vi "Position Heading.vi"(10 "To":T2, 11 "From":T2) -> (2 "Same Position?":bool, 3 "Heading":T1)   [LabVIEW 2020, in "SquareBattle.lvlib"]
doc: "Returns the closest direction enumeration value from the specified From position to the specied To position. This can be used to more easily move towards a goal position.\n\nIf Same Position? returns True, then the To and From positions are the same and the Heading output will be invalid."
uses:
  SquareBattle.lvlib
  Position.ctl
  Direction.ctl
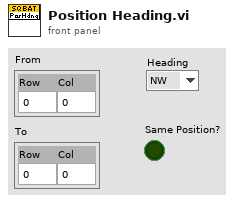
[diagram p1: front panel]
types:
  T1 = typedef "SquareBattle.lvlib/Direction.ctl" = enum16{"NW", "N", "NE", "E", "SE", "S", "SW", "W"}
  T2 = typedef "SquareBattle.lvlib/Position.ctl" = cluster{"Row":i32, "Col":i32}
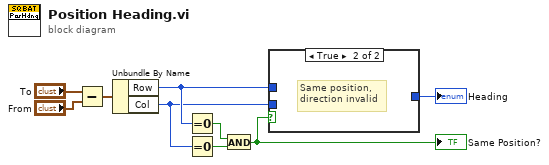
[diagram p0: block diagram]
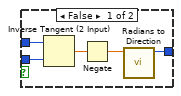
[diagram p2: hidden frame]
diagram:
  n1 = Subtract(x="To", y="From") -> (x-y=w6:T2)
  n2 = Unbundle By Name(w6) -> ("Row"=w5:i32, "Col"=w4:i32)
  n3 = Equal To 0?(x=w5) -> (x = 0?=w3:bool)
  n4 = Equal To 0?(x=w4) -> (x = 0?=w2:bool)
  n5 = And(x=w3, y=w2) -> (x .and. y?=w1:bool)
  "Same Position?" <- w1
  n6 = case shown="True" w1 {
    tunnel: [w12 _] -> w7
    tunnel: w5 -> [w11 _]
    tunnel: w4 -> [w10 _]
    frame False {
      n7 = Inverse Tangent (2 Input)(1:w10, 2:w11) -> (0:w14:dbl)
      n8 = Negate(x=w14) -> (-x=w13:dbl)
      n9 = call "Radians to Direction.vi"("Radian Heading (0 = East)"=w13) -> ("Closest Direction"=w12:T1)  [unwired: 10 in]
    }
    frame True {
      # "Same position,\ndirection invalid"
    }
  }
  "Heading" <- w7
